vi "Tosca-Get Multirig Config Table.vi"(7 "Rigs":string[](array[string])) -> (8 "Table":T1(array[cluster]))   [LabVIEW 2020]
uses:
  epl-vi-lib/Utility VIs/File IO VIs/Configuration File Wrapper VIs/Config-Read Key (string).vi
  epl-vi-lib/Utility VIs/Type Defs/TCP Params.ctl
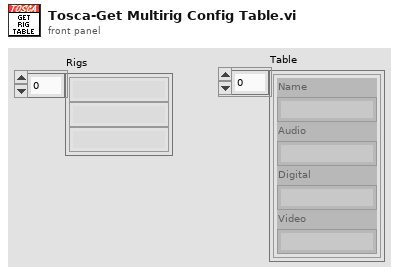
[diagram p1: front panel]
types:
  T1 = cluster{"Name":string, "Audio":string, "Digital":string, "Video":string}[]
  T2 = typedef "TCP Params.ctl" = cluster{"IP Address":string, "Port":i32}
  T3 = cluster{"String":string, "value":string, "value":string, "Address out":string}
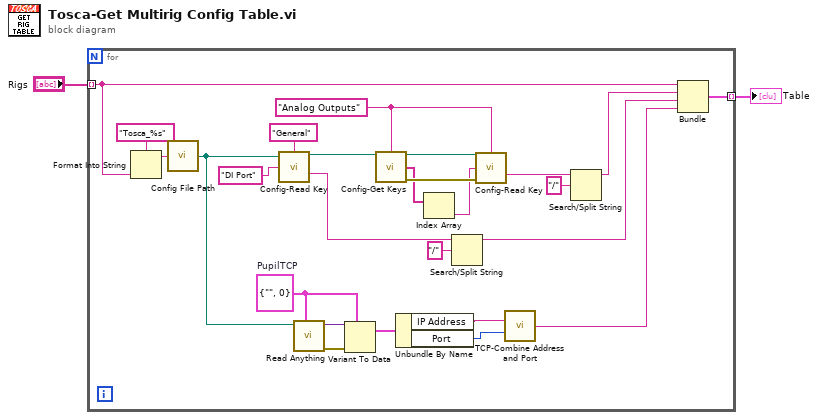
[diagram p0: block diagram]
diagram:
  n1 = for {
    tunnel: "Rigs" -> [w26] mode=indexing
    tunnel: [w25] -> w1 mode=indexing
    w7 = T2 {"IP Address"="", "Port"=0}  # PupilTCP
    w14 = "Analog Outputs" ("section")
    n2 = Format Into String(format string="Tosca_%s", w26) -> (resulting string=w27:string)  [unwired: 2 in, 1 out]
    n3 = call "Config File Path.vi"("AppName"=w27) -> ("Default config file name"=w6:path)
    n4 = call-poly "Config-Read Key.vi"("configuration file path"=w6, "section"="General", "key"="DI Port") -> ("file path"=w17:path, "value"=w20:string)  [unwired: 9 in, 2 out]
    n5 = call "Read Anything.vi"("Type of Anything"=w7, "Path (dialog)"=w6) -> ("Error Out"=w9:errorcluster, "Anything"=w8:variant)  [unwired: 7 in, 1 out]
    n6 = Variant To Data(error in=w9, type=w7, Variant=w8) -> (data=w10:T2)  [unwired: 1 out]
    n7 = call "Config-Get Keys.vi"("configuration file path"=w17, "section"=w14) -> ("file path"=w16:path, "key names"=w13:string[], "error out"=w15:errorcluster)  [unwired: 11 in]
    n8 = Unbundle By Name(w10) -> ("IP Address"=w5:string, "Port"=w4:i32)
    n9 = Index Array(array=w13) -> (element=w12:string)  [unwired: 1 in]
    n10 = Search/Split String(string=w20, search string/char (-)="/") -> (substring before match=w24:string)  [unwired: 1 in, 2 out]
    n11 = call-poly "Config-Read Key.vi"("configuration file path"=w16, "section"=w14, "key"=w12, "error in (no error)"=w15) -> ("value"=w11:string)  [unwired: 8 in, 3 out]
    n12 = call "TCP-Combine Address and Port.vi"("Address"=w5, "Port"=w4) -> ("Address out"=w3:string)  [unwired: 13 in]
    n13 = Search/Split String(string=w11, search string/char (-)="/") -> (substring before match=w18:string)  [unwired: 1 in, 2 out]
    n14 = Bundle("String"=w26, "value"=w18, "value"=w24, "Address out"=w3) -> (w25:T3)  [unwired: 1 in]
  }
  "Table" <- w1
